vi "LED GLOBALS!!!.vi"() -> ()   [LabVIEW 2020]
uses:
  LED_Control_States.ctl
panel:
  in  "Numbers":dbl[](array[numeric])=[2.0, 4.0, 100.0, 30.0, 2.0, 6.0]
  in  "colors":u32[](array[colorbox])=[16712704, 1507583, 65302]
  in  "Nya :3 Control_State  4":T1=enum."swapperlines"
  in  "Nya :3 Control_State 3":T1=enum."swapperlines"
  in  "Nya :3 Control_State  2":T1=enum."swapperlines"
  in  "Nya :3 Control_State":T1=enum."swapperlines"
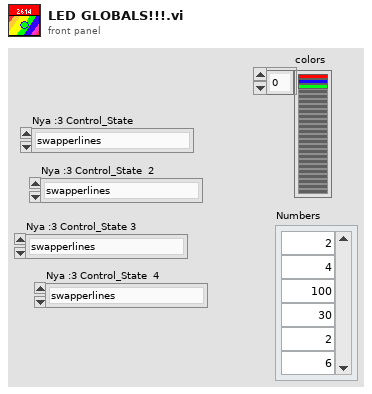
[diagram p1: front panel]
types:
  T1 = typedef "LED_Control_States.ctl" = enum16{"Config-Stripes", "swapperlines", "Rand", "Solid", "Flash-S", "Gradyent", "Move-Stripes", "Org-Rand", "Move-Point-Tail", "Flames", "Fade", "Alt-Colors"}
diagram:
